vi "Write Text (Variant).vi"(8 "error in":errorcluster, 10 "Anything":variant, 11 "file in":refnum<file>) -> (0 "error out":errorcluster, 3 "file out":refnum<file>)   [LabVIEW 2021, in "Diagnostics.lvlib"]
doc: "Write a variant as XML to the debug log file."
uses:
  Diagnostics.lvlib
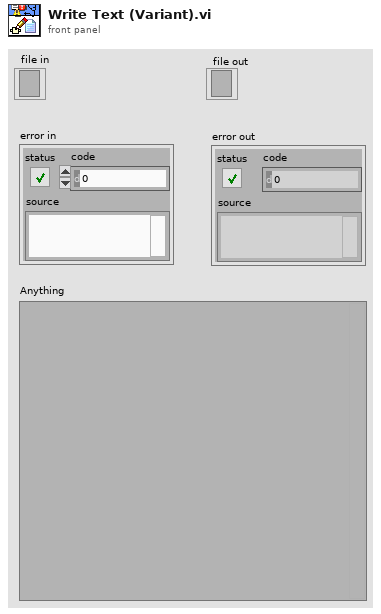
[diagram p1: front panel]
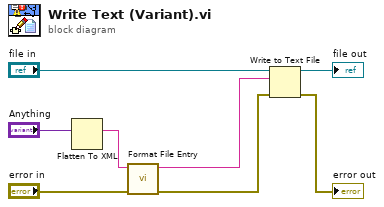
[diagram p0: block diagram]
diagram:
  n1 = Flatten To XML(6:"Anything") -> (2:w1:string)
  n2 = call "Format File Entry.vi"("error in (no error)"="error in", "message"=w1) -> ("error out"=w2:errorcluster, "formatted string"=w4:string)  [unwired: 8 in]
  n3 = Write to Text File(file (use dialog)="file in", text=w4, error in=w2) -> (refnum out=→"file out":refnum<file>, error out=→"error out":errorcluster)  [unwired: 1 in, 1 out]
